vi "GEOM_Convert2detheaders_NOAO.vi"(4 "single headers":string[][](array[string]), 6 "detsize":string[](array[string]), 8 "Binning":T1={"x"=1, "y"=1} {"y" min=1; "x" min=1}, 9 "ME Headers in":string[][][](array[string]), 10 "detectors":T2[](array[typedef]), 11 "detext":bool) -> (1 "ME Headers out":string[][][](array[string]))   [LabVIEW 2016]
uses:
  GEOM_DetSummaryStruct.ctl
  GEOM_Binning.ctl
panel:
  in  "Corrected ROI":T3={"xstart"=1, "ystart"=1, "xsize"=1, "ysize"=1}
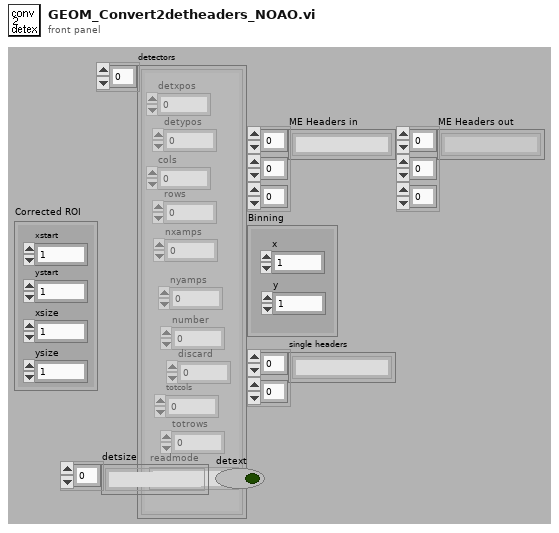
[diagram p1: front panel]
types:
  T1 = typedef "GEOM_Binning.ctl" = cluster{"x":u32, "y":u32}
  T2 = typedef "GEOM_DetSummaryStruct.ctl" = cluster{"detxpos":i32, "detypos":i32, "cols":i32, "rows":i32, "nxamps":i32, "nyamps":i32, "number":i32, "discard":i32, "totcols":i32, "totrows":i32, "readmode":string}
  T3 = cluster{"xstart":u32, "ystart":u32, "xsize":u32, "ysize":u32}
  T4 = cluster{"xstart":u32, "ystart":u32, "xsize":u32, "ysize":u32}[]
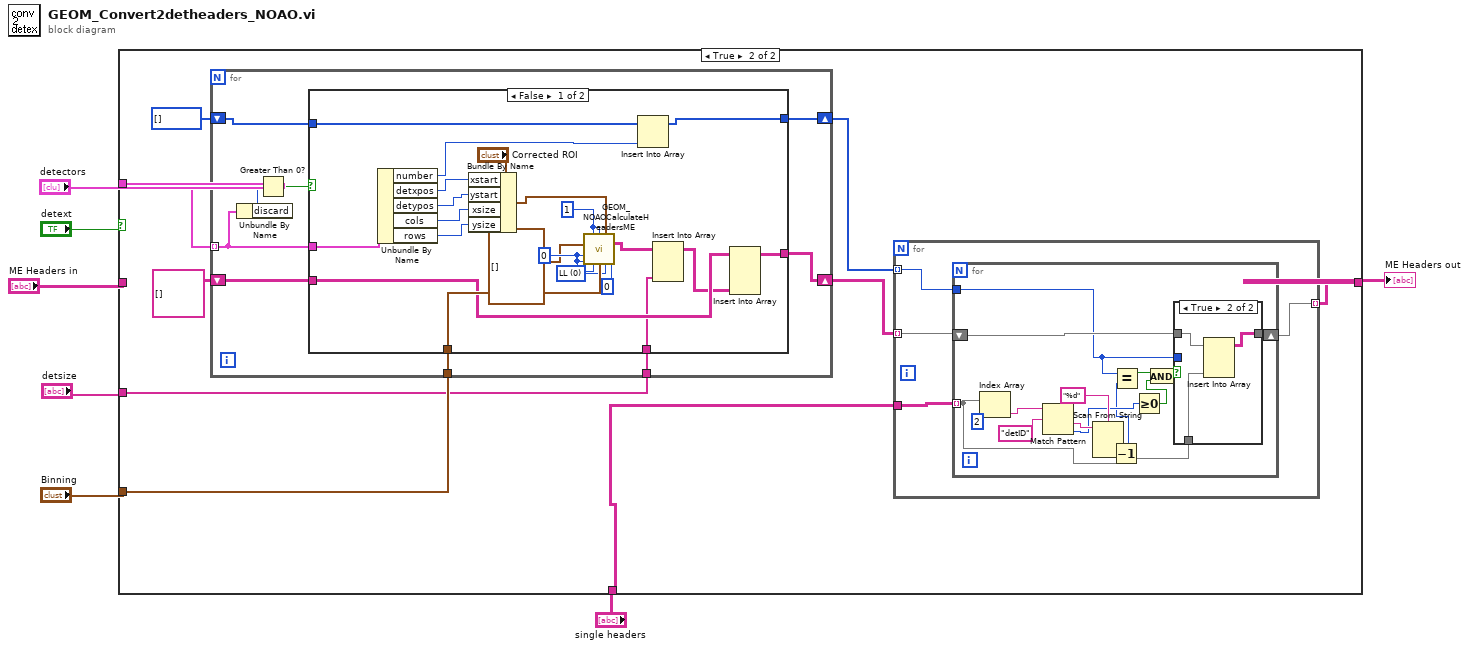
[diagram p0: block diagram]
diagram:
  n1 = case shown="True" "detext" {
    tunnel: "ME Headers in" -> [w8 _]
    tunnel: [w8 w13] -> w2
    tunnel: "detectors" -> [_ w14]
    tunnel: "single headers" -> [_ w17]
    tunnel: "Binning" -> [_ w16]
    tunnel: "detsize" -> [_ w15]
    frame False {
    }
    frame True {
      n2 = for {
        tunnel: w16 -> [w26]
        tunnel: w15 -> [w25]
        tunnel: w14 -> [w22] mode=indexing
        shift-right: [w24] -> w12
        shift-left: string[][][] [] ("ME Headers out") -> [w23]
        shift-right: [w19] -> w9
        shift-left: i32[] [] -> [w18]
        n3 = Unbundle By Name(w22) -> ("discard"=w21:i32)
        n4 = Greater Than 0?(x=w21) -> (x > 0?=w20:bool)
        n5 = case shown="False" w20 {
          tunnel: w26 -> [w47 _]
          tunnel: w25 -> [w32 _]
          tunnel: w22 -> [w46 _]
          tunnel: [w30 w49] -> w24
          tunnel: w23 -> [w34 w49]
          tunnel: [w28 w48] -> w19
          tunnel: w18 -> [w27 w48]
          frame False {
            w44 = u16 0 items=["LL", "LR", "UL", "UR"] ("type")
            w41 = 1 ("ampxstart")
            w45 = 0 ("overscan")
            n6 = Unbundle By Name(w46) -> ("number"=w29:i32, "detxpos"=w39:i32, "detypos"=w38:i32, "cols"=w37:i32, "rows"=w36:i32)
            n7 = Bundle By Name(cluster="Corrected ROI", "xstart"=w39, "ystart"=w38, "xsize"=w37, "ysize"=w36) -> (w35:T3)
            n8 = call "GEOM_NOAOCalculateHeadersME.vi"("ampxstart"=w41, "ampystart"=w41, "Corrected ROI"=w35, "Requested ROIs"=T4 [], "overscan"=w45, "trims"=w45, "bias skip begining"=w45, "Binning"=w47, "type"=w44, "ytrims"=0) -> ("ME Headers out"=w33:string[][])  [unwired: 3 in, 2 out]
            n9 = Insert Into Array(array=w27, new element=w29) -> (w28:i32[])  [unwired: 1 in]
            n10 = Insert Into Array(array=w33, new element=w32) -> (w31:string[][])  [unwired: 2 in]
            n11 = Insert Into Array(array=w34, new element=w31) -> (w30:string[][][])  [unwired: 3 in]
          }
          frame True {
          }
        }
      }
      n12 = for {
        tunnel: w17 -> [w53]
        tunnel: [w52] -> w13 mode=indexing
        tunnel: w12 -> [w51] mode=indexing
        tunnel: w9 -> [w50] mode=indexing
        n13 = for {
          tunnel: w53 -> [w61] mode=indexing
          shift-right: [w59] -> w52
          shift-left: w51 -> [w60]
          tunnel: w50 -> [w54]
          n14 = Index Array(array=w61, index=2) -> (element=w67:string)
          n15 = Match Pattern(string=w67, regular expression="detID") -> (after substring=w65:string, offset past match=w57:i32)  [unwired: 3 out]
          n16 = Scan From String(format string="%d", input string=w65) -> (output 1=w63:i32)  [unwired: 2 in, 4 out]
          n17 = Decrement(x=w63) -> (x-1=w55:i32)
          n18 = Equal?(x=w54, y=w55) -> (x = y?=w62:bool)
          n19 = Greater Or Equal To 0?(x=w57) -> (x >= 0?=w56:bool)
          n20 = And(x=w62, y=w56) -> (x .and. y?=w58:bool)
          n21 = case shown="True" w58 {
            tunnel: w61 -> [_ w70]
            tunnel: w60 -> [w69 w72]
            tunnel: [w69 w71] -> w59
            tunnel: w54 -> [_ _]
            frame False {
            }
            frame True {
              n22 = Insert Into Array(array=w72, new element=w70) -> (w71:string[][])  [unwired: 2 in]
            }
          }
        }
      }
    }
  }
  "ME Headers out" <- w2
